vi "make_installer_exe.vi"(4 "config_value":T2, 6 "config_include":T1, 8 "error in (no error)":errorcluster, 10 "installer_directory":path, 11 "setup_filename in":path) -> (0 "error out":errorcluster, 3 "setup_filename out":path)   [LabVIEW 2015, in "lv-bin-7zip.lvlib"]
uses:
  lv-bin-7zip.lvlib
  <userlib>/antonio-alexander/lv-bin/public/api/v1/v1.lvlib
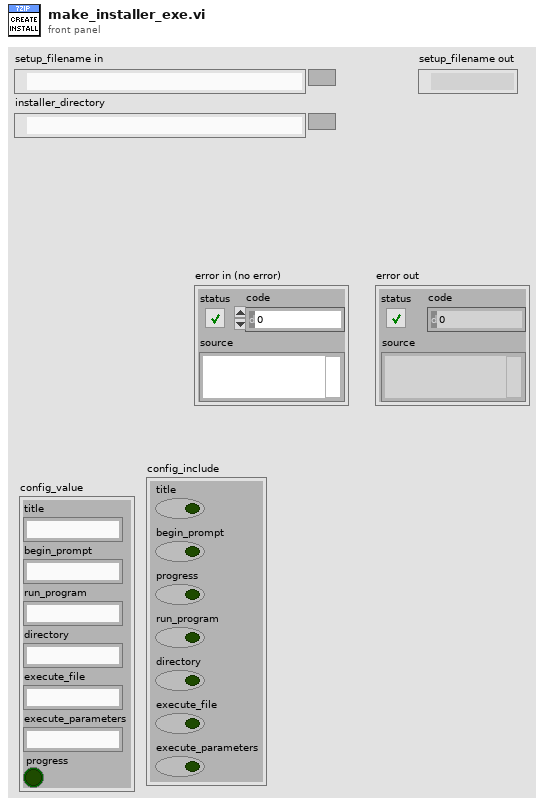
[diagram p1: front panel]
types:
  T1 = cluster{"title":bool, "begin_prompt":bool, "progress":bool, "run_program":bool, "directory":bool, "execute_file":bool, "execute_parameters":bool}
  T2 = cluster{"title":string, "begin_prompt":string, "run_program":string, "directory":string, "execute_file":string, "execute_parameters":string, "progress":bool}
  T3 = typedef "lv-bin.lvlib/v1.lvlib/temp_dir_config.ctl" = cluster{"root_folder":path, "prefix":string}
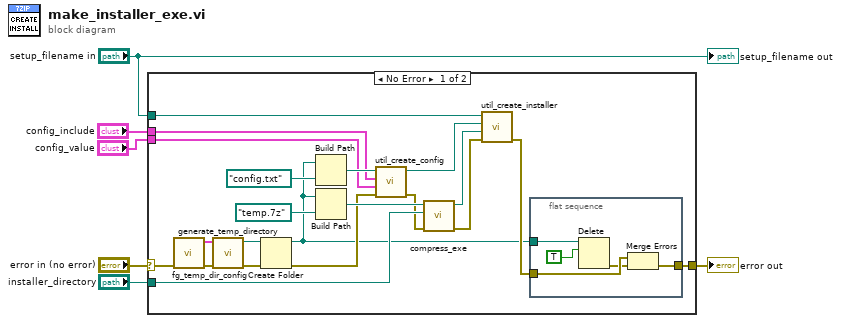
[diagram p0: block diagram]
diagram:
  n1 = case shown="No Error" "error in (no error)" {
    selector: "error in (no error)" -> [w7 w33]
    tunnel: "installer_directory" -> [w25 _]
    tunnel: "setup_filename in" -> [w15 _]
    tunnel: [w13 w33] -> w2
    tunnel: "config_include" -> [w19 _]
    tunnel: "config_value" -> [w18 _]
    frame No Error {
      n2 = call "fg_temp_dir_config.vi"("error in (no error)"=w7) -> ("error out"=w8:errorcluster, "temp_dir_config out"=w9:T3)  [unwired: 9 in]
      n3 = call <userlib>:"generate_temp_directory.vi"("error in (no error)"=w8, "configuration"=w9) -> ("error out"=w17:errorcluster, "temp_dir"=w16:path)  [unwired: 8 in]
      n4 = Create Folder(path (use dialog)=w16, error in=w17) -> (created path=w10:path, error out=w12:errorcluster)  [unwired: 1 in, 1 out]
      n5 = Build Path(base path=w10, name or relative path=path "config.txt" ("Path in (Relative)")) -> (appended path=w23:path)
      n6 = Build Path(base path=w10, name or relative path=path "temp.7z" ("Path in (Relative)")) -> (appended path=w26:path)
      n7 = call "util_create_config.vi"("error in (no error)"=w12, "config_value"=w18, "config_include"=w19, "config_file in"=w23) -> ("error out"=w11:errorcluster, "config_file out"=w21:path)  [unwired: 6 in]
      n8 = call "compress_exe.vi"("error in (no error)"=w11, "files_to_add"=w25, "archive_path in"=w26) -> ("error out"=w22:errorcluster, "archive_path out"=w20:path)  [unwired: 7 in]
      n9 = call "util_create_installer.vi"("error in (no error)"=w22, "archive"=w20, "config"=w21, "install_file in"=w15) -> ("error out"=w14:errorcluster)  [unwired: 6 in, 1 out]
      n10 = flat-sequence {
        tunnel: w10 -> [w32]
        tunnel: w14 -> [w30]
        tunnel: [w28] -> w13
        frame #0 {
          n11 = Delete(path (use dialog)=w32, entire hierarchy (F)=TRUE) -> (error out=w29:errorcluster)  [unwired: 3 in, 2 out]
          n12 = Merge Errors(w30, w29) -> (w28:errorcluster)
        }
      }
    }
    frame Error {
    }
  }
  "error out" <- w2
  "setup_filename out" <- "setup_filename in"
